vi "Redraw Colours.vi"(8 "error in (no error)":errorcluster, 11 "Graph Manager in":refnum<class "Graph Manager.lvclass">) -> (0 "error out":errorcluster, 3 "Graph Manager out":refnum<class "Graph Manager.lvclass">)   [LabVIEW 2016, in "Graph Manager.lvclass"]
uses:
  Graph Manager.lvclass
  Graph Manager.lvclass/Graph Manager.ctl
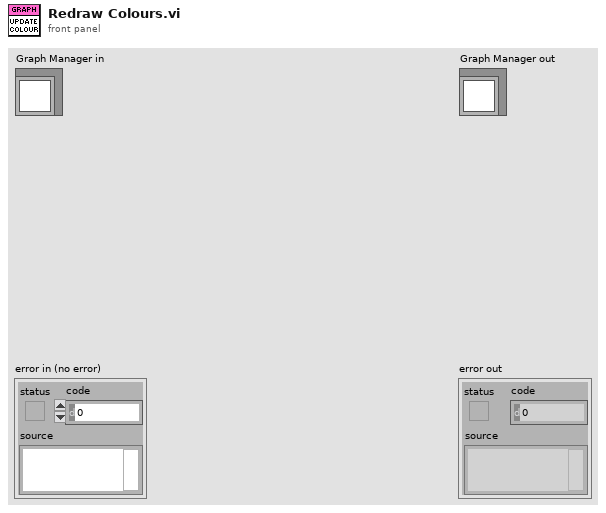
[diagram p1: front panel]
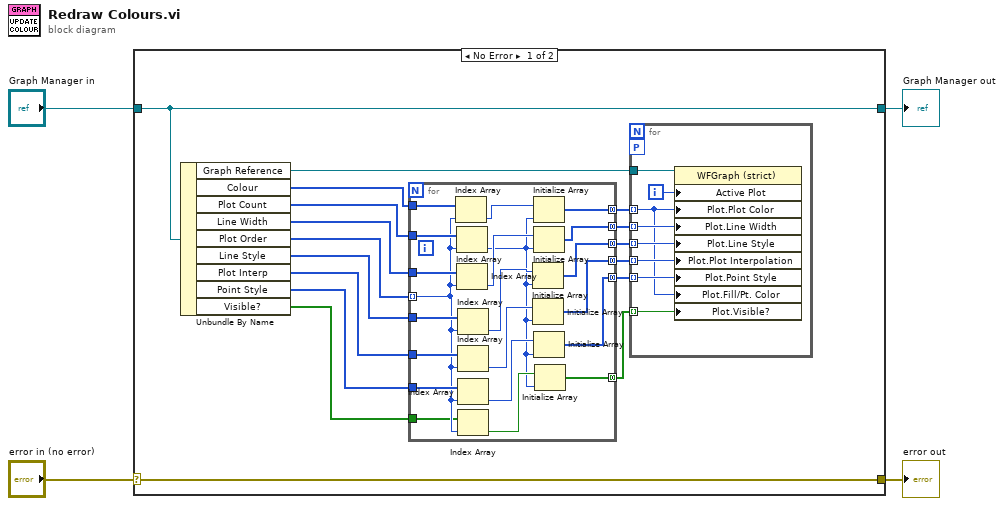
[diagram p0: block diagram]
diagram:
  n1 = case shown="No Error" "error in (no error)" {
    selector: "error in (no error)" -> [w21 w52]
    tunnel: [w21 w52] -> w3
    tunnel: [w20 w51] -> w1
    tunnel: "Graph Manager in" -> [w20 w51]
    frame No Error {
      n2 = Unbundle By Name(w20) -> ("Graph Reference"=w19:refnum<vi>, "Colour"=w18:u32[], "Plot Count"=w13:i32[], "Line Width"=w15:u8[], "Plot Order"=w14:i32[], "Line Style"=w12:u8[], "Plot Interp"=w11:u8[], "Point Style"=w10:u8[], "Visible?"=w6:bool[])
      n3 = for {
        tunnel: w18 -> [w41]
        tunnel: [w42] -> w17 mode=concatenating
        tunnel: [w37] -> w16 mode=concatenating
        tunnel: w15 -> [w39]
        tunnel: w14 -> [w26] mode=indexing
        tunnel: w13 -> [w36]
        tunnel: w12 -> [w35]
        tunnel: w11 -> [w34]
        tunnel: w10 -> [w33]
        tunnel: [w29] -> w9 mode=concatenating
        tunnel: [w28] -> w8 mode=concatenating
        tunnel: [w27] -> w7 mode=concatenating
        tunnel: w6 -> [w23]
        tunnel: [w22] -> w5 mode=concatenating
        n4 = Index Array(array=w41, index=w26) -> (element=w40:u32)
        n5 = Index Array(array=w36, index=w26) -> (element=w24:i32)
        n6 = Index Array(array=w39, index=w26) -> (element=w38:u8)
        n7 = Index Array(array=w35, index=w26) -> (element=w32:u8)
        n8 = Index Array(array=w34, index=w26) -> (element=w31:u8)
        n9 = Index Array(array=w33, index=w26) -> (element=w30:u8)
        n10 = Index Array(array=w23, index=w26) -> (element=w25:bool)
        n11 = Initialize Array(w32, w24) -> (w29:u8[])
        n12 = Initialize Array(w31, w24) -> (w28:u8[])
        n13 = Initialize Array(w40, w24) -> (w42:u32[])
        n14 = Initialize Array(w38, w24) -> (w37:u8[])
        n15 = Initialize Array(w30, w24) -> (w27:u8[])
        n16 = Initialize Array(w25, w24) -> (w22:bool[])
      }
      n17 = for {
        tunnel: w19 -> [w50]
        workers-P: _ -> [_]
        tunnel: w17 -> [w44] mode=indexing
        tunnel: w16 -> [w48] mode=indexing
        tunnel: w9 -> [w47] mode=indexing
        tunnel: w8 -> [w46] mode=indexing
        tunnel: w7 -> [w45] mode=indexing
        tunnel: w5 -> [w43] mode=indexing
        i -> [w49]
        n18 = property class="WFGraph (strict)"(reference=w50, "Active Plot"=w49, "Plot.Plot Color"=w44, "Plot.Line Width"=w48, "Plot.Line Style"=w47, "Plot.Plot Interpolation"=w46, "Plot.Point Style"=w45, "Plot.Fill/Pt. Color"=w44, "Plot.Visible?"=w43) -> ()  [unwired: 1 in, 2 out]
      }
    }
    frame Error {
    }
  }
  "error out" <- w3
  "Graph Manager out" <- w1
